vi "SMO.jsonRPC.Process.vi"(8 "error in (no error)":errorcluster, 11 "SMO.jsonRPC in":refnum<class "SMO.jsonRPC.lvclass">) -> (0 "error out":errorcluster)   [LabVIEW 2013, in "SMO.jsonRPC.lvclass"]
uses:
  SMO.jsonRPC.lvclass
  Typedefs/Request--Cluster.ctl
  <vilib>/JKI/JKI JSON RPC Specification/Request/Request.lvclass
  <vilib>/JKI/JKI JSON RPC Specification/Response/Response.lvclass
  <vilib>/JKI/JKI SMO/SMO/SMO.lvclass
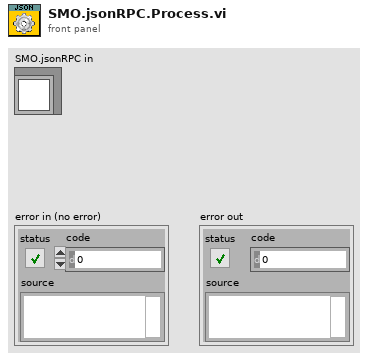
[diagram p1: front panel]
types:
  T1 = enum32{"invalid app kind", "Development System", "Run Time System", "Student Edition", "Embedded LabVIEW", "Evaluation", "Custom"}
  T2 = cluster{"Current VI Reference":refnum<vi>, "Close Panel on Exit?":bool, "error":errorcluster, "Standalone":bool}
  T3 = enum32{"Invalid", "Standard", "Closed", "Hidden", "Minimized", "Maximized"}
  T4 = typedef "SMO.jsonRPC.lvclass/Request--Cluster.ctl" = cluster{"Request":refnum<class "Request.lvclass">, "reply queue":refnum<queue>, "Async?":bool}
  T5 = cluster{"Core":cluster{"Current VI Reference":refnum<vi>, "Close Panel on Exit?":bool, "error":errorcluster, "Standalone":bool}, "Self Reference":refnum<class "SMO.jsonRPC.lvclass">, "Message Payload":T4}
  T6 = typedef "SMO.lvclass/SMOState --Enum.ctl" = enum16{"unknown", "Created", "Started", "Stopped"}
  T7 = typedef "SMO.lvclass/Protected Events.ctl" = cluster{"StopProcesses":refnum<user-event>, "AbortProcesses":refnum<user-event>, "Config Changed":refnum<user-event>}
  T8 = typedef "SMO.jsonRPC.lvclass/PrivateEvents--Cluster.ctl" = cluster{"Incoming Request":refnum<user-event>}
  T9 = typedef "SMO.jsonRPC.lvclass/PublicEvents--Cluster.ctl" = cluster{"Reply":refnum<user-event>}
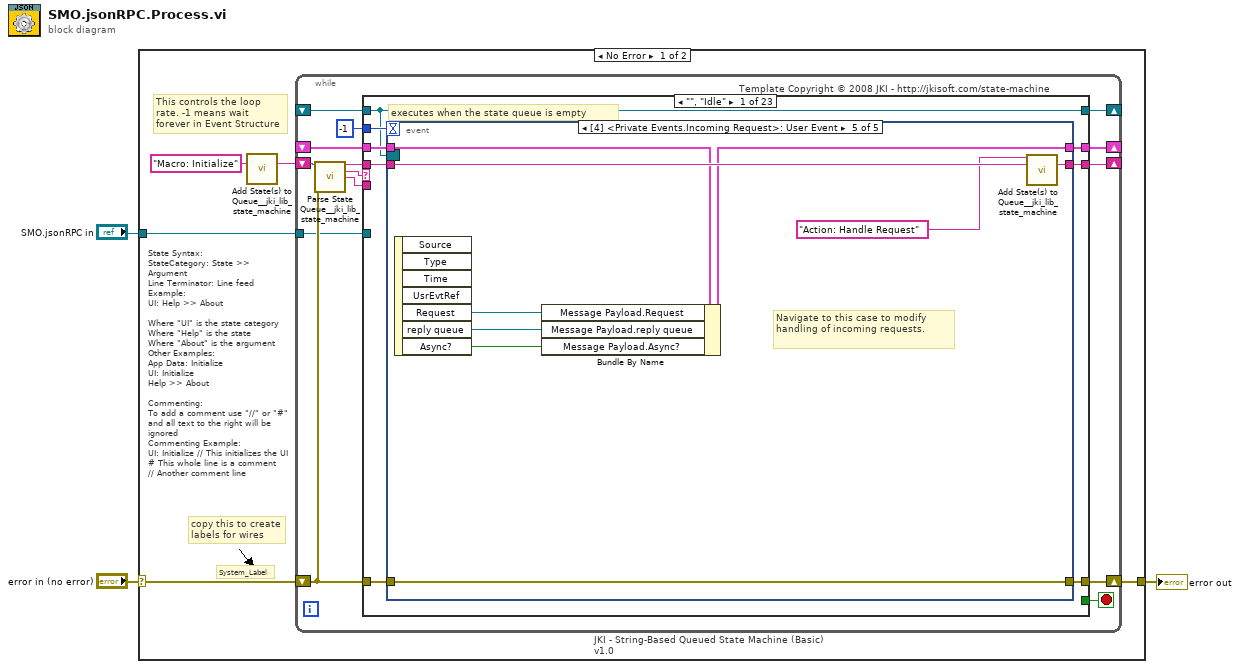
[diagram p0: block diagram]
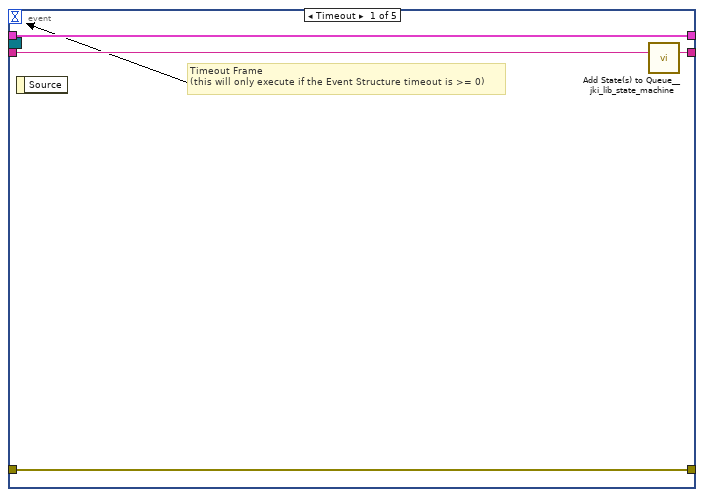
[diagram p2: hidden frame]
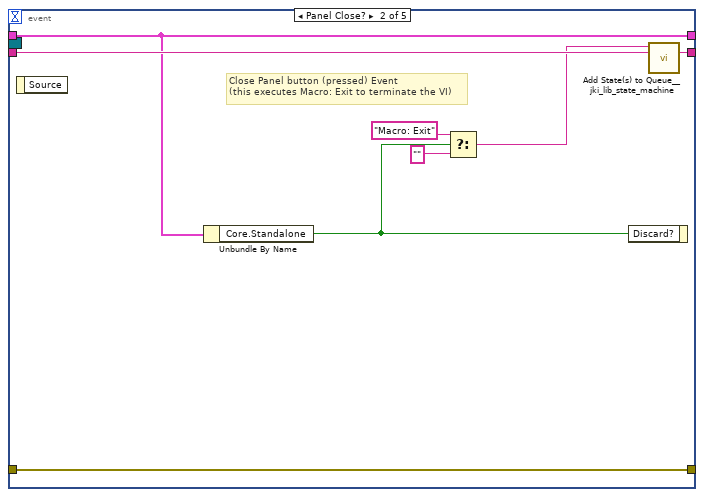
[diagram p3: hidden frame]
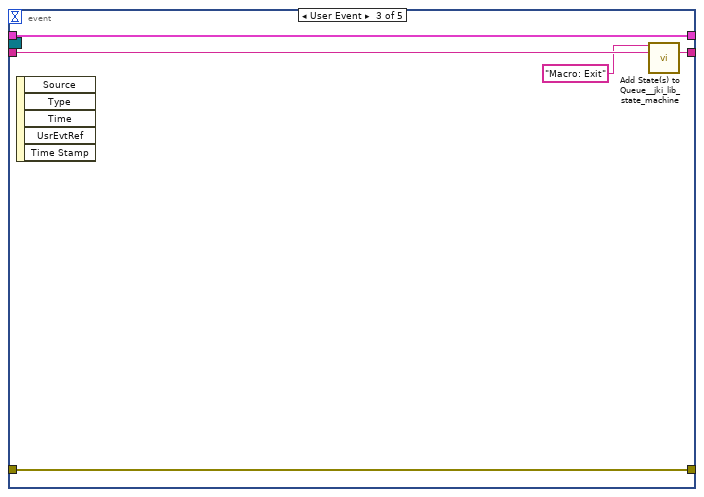
[diagram p4: hidden frame]
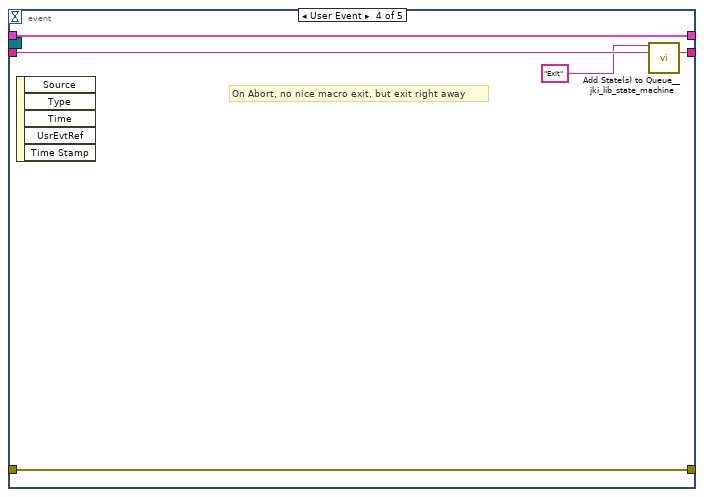
[diagram p5: hidden frame]
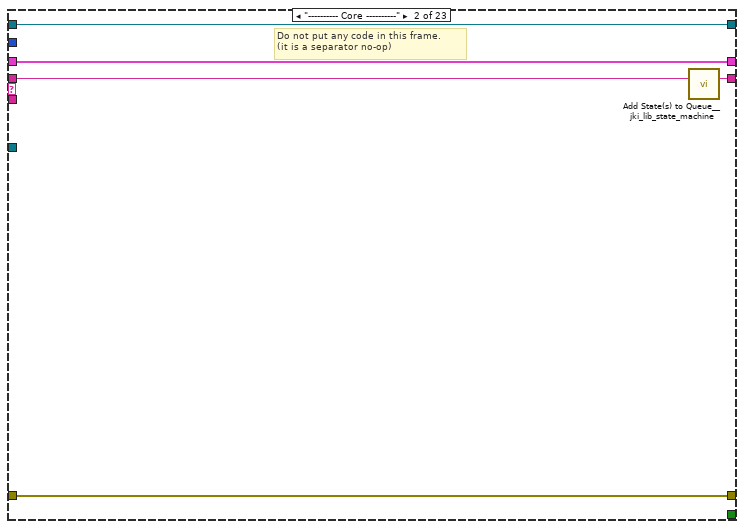
[diagram p6: hidden frame]
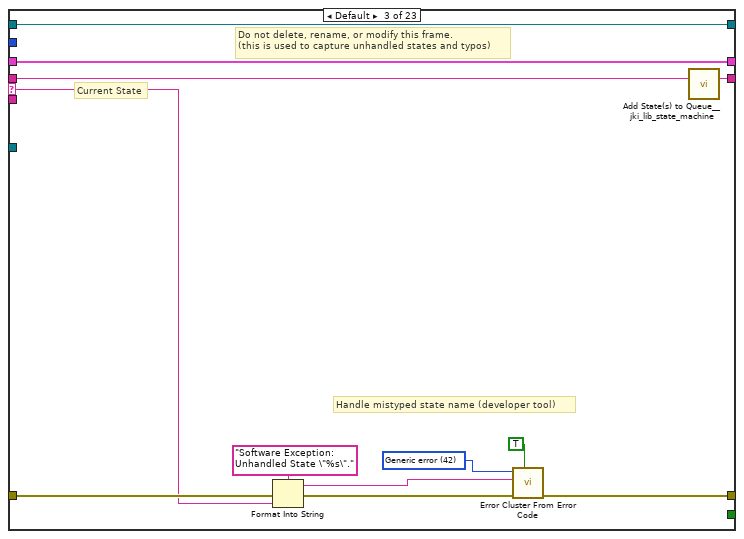
[diagram p7: hidden frame]
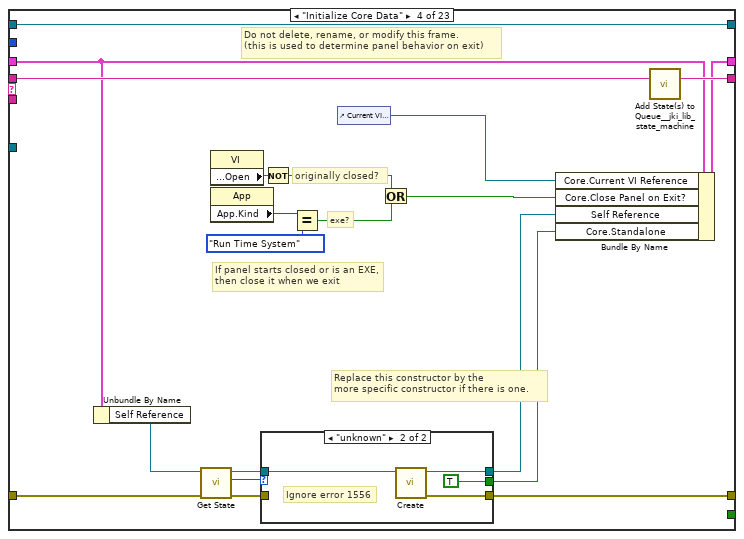
[diagram p8: hidden frame]
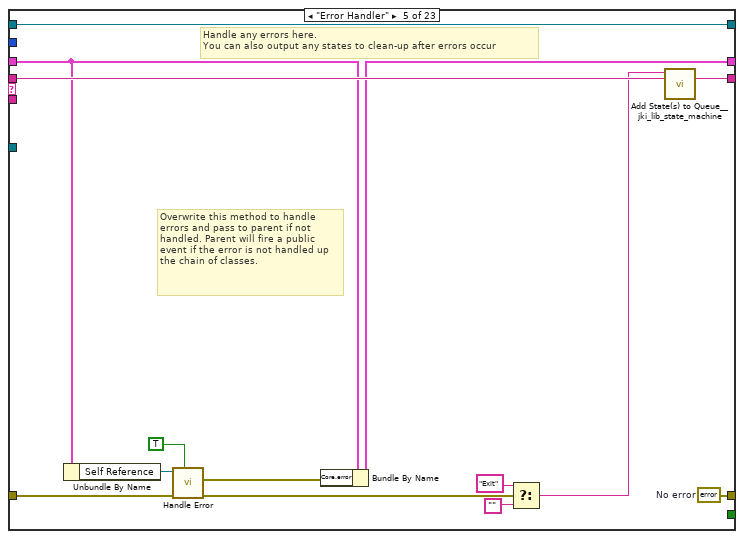
[diagram p10: hidden frame]
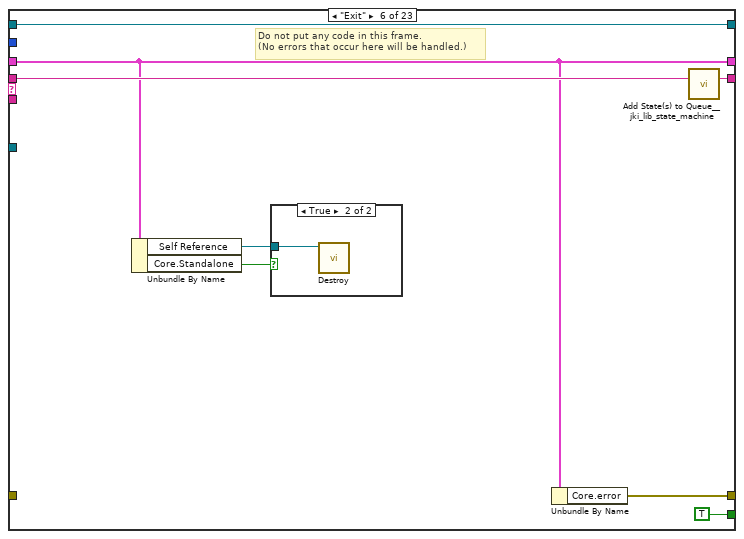
[diagram p11: hidden frame]
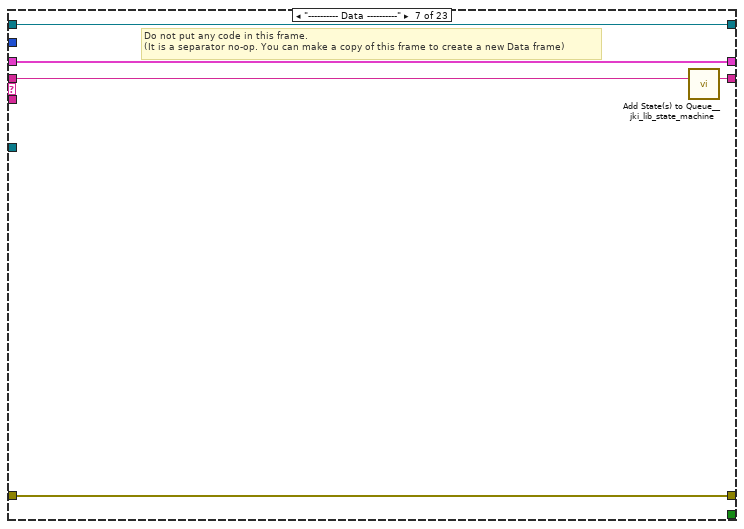
[diagram p13: hidden frame]
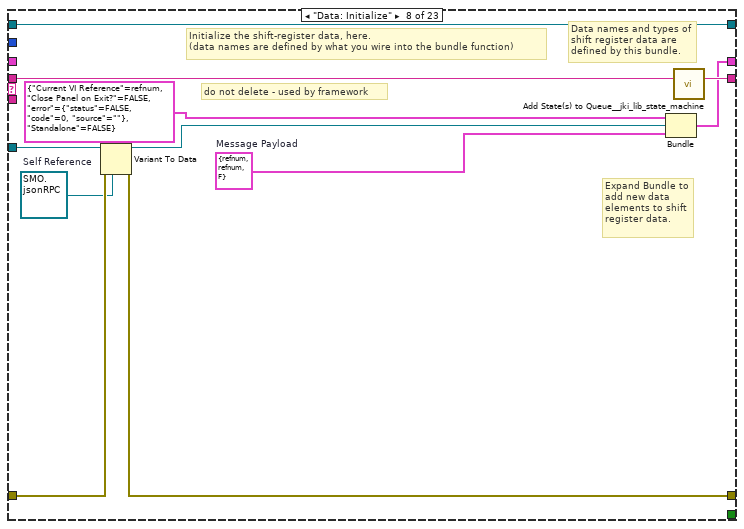
[diagram p14: hidden frame]
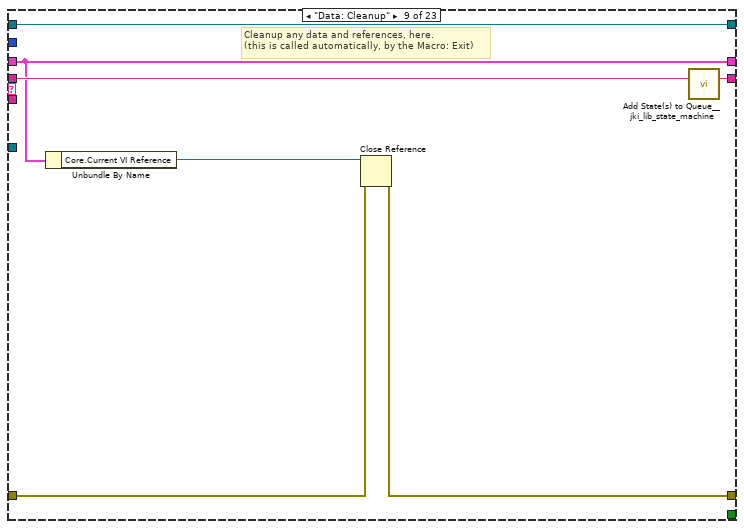
[diagram p15: hidden frame]
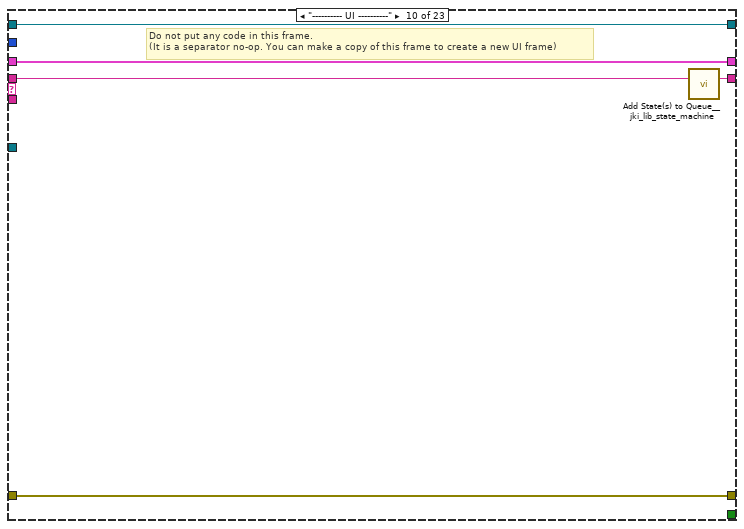
[diagram p16: hidden frame]
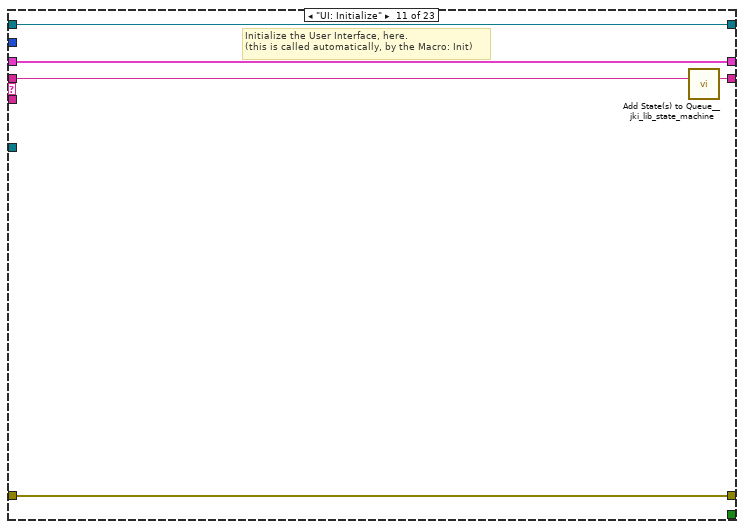
[diagram p17: hidden frame]
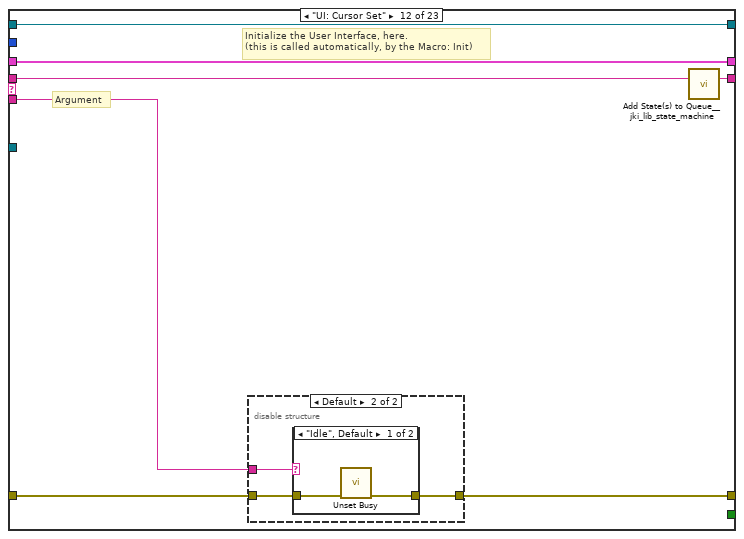
[diagram p18: hidden frame]
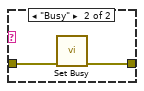
[diagram p20: hidden frame]
diagram:
  n1 = case shown="No Error" "error in (no error)" {
    selector: "error in (no error)" -> [w5 w304]
    tunnel: "SMO.jsonRPC in" -> [w6 _]
    tunnel: [w4 w304] -> w3
    frame No Error {
      # "State Syntax:\nStateCategory: State >> Argument\nLine Terminator: Line feed\nExample:\nUI: Help >> About\n\nWhere \"UI\" is the state category\nWhere \"Help\" is the state\nWhere \"About\" is the argument\nOther Examples:\nApp Data: Initialize\nUI: Initialize\nHelp >> About\n\nCommenting:\nTo add a comment use \"//\" or \"#\" and all text to the right will be ignored\nCommenting Example:\nUI: Initialize // This initializes the UI\n# This whole line is a comment\n// Another comment line"
      # "copy this to create labels for wires"
      # "This controls the loop rate. -1 means wait forever in Event Structure"
      # "System_Label"
      n2 = call <vilib>:"Add State(s) to Queue__jki_lib_state_machine.vi"("State(s) in (\"\")"="Macro: Initialize") -> ("States Out"=w8:string)  [unwired: 14 in]
      n3 = while "JKI - String-Based Queued State Machine (Basic) v1.0" {
        shift-right: [w15] -> _
        shift-left: _ -> [w14]
        shift-right: [w18] -> w4
        shift-left: w5 -> [w12]
        shift-right: [w17] -> _
        shift-left: w8 -> [w19]
        tunnel: w6 -> [w11]
        shift-right: [w10] -> _
        shift-left: _ -> [w9]
        stop <- w16 stop-if-true
        # "Template Copyright © 2008 JKI - http://jkisoft.com/state-machine"
        n4 = call <vilib>:"Parse State Queue__jki_lib_state_machine.vi"("State Queue"=w19, "Error In (no error)"=w12) -> ("Remaining States"=w21:string, "Current State"=w22:string, "Arguments"=w20:string)  [unwired: 11 in]
        n5 = case shown="\"\", \"Idle\"" w22 {
          selector: w22 -> [_ _ w68 _ _ _ _ _ _ _ _ _ _ _ _ _ _ _ _ _ _ _ _]
          tunnel: w21 -> [w30 w66 w72 w98 w118 w126 w132 w143 w150 w155 w160 w167 w183 w215 w221 w232 w237 w246 w259 w272 w278 w283 w299]
          tunnel: w20 -> [_ _ _ _ _ _ _ _ _ _ _ w161 w177 _ _ _ _ _ _ _ _ _ _]
          tunnel: w14 -> [w28 w63 w70 w82 w107 w119 w129 _ w145 w152 w158 w165 w179 w212 w217 w223 w234 w243 w256 w270 w276 w281 w296]
          tunnel: [w27 w64 w74 w81 w109 w122 w130 w139 w146 w153 w157 w162 w180 w213 w219 w230 w235 w240 w257 w260 w274 w279 w285] -> w18
          tunnel: w12 -> [w26 w64 w73 w83 w114 _ w130 w140 w147 w153 w157 w163 w181 w213 w219 w230 w235 w241 w257 w264 w274 w279 w294]
          tunnel: [w29 w65 w71 w97 w117 w125 w131 w142 w149 w154 w159 w166 w182 w214 w220 w231 w236 w245 w258 w271 w277 w282 w298] -> w17
          tunnel: [_ _ _ _ _ TRUE _ _ _ _ _ _ _ _ _ _ _ _ _ _ _ _ _] -> w16
          tunnel: [w25 w63 w70 w96 w106 w119 w129 w141 w145 w152 w158 w165 w179 w212 w217 w223 w234 w243 w256 w270 w276 w281 w296] -> w15
          tunnel: -1 ("Timeout") -> [w24 _ _ _ _ _ _ _ _ _ _ _ _ _ _ _ _ _ _ _ _ _ _]
          tunnel: w11 -> [_ _ _ _ _ _ _ w137 _ _ _ _ _ _ _ _ _ _ _ _ _ _ _]
          tunnel: [w23 w62 w67 w89 w116 w123 w128 w135 w144 w151 w156 w164 w176 w211 w218 w224 w233 w244 w255 w269 w275 w280 w297] -> w10
          tunnel: w9 -> [w23 w62 w67 w89 w116 w123 w128 w135 w144 w151 w156 w164 w176 w211 w218 w224 w233 w244 w255 _ w275 w280 w297]
          frame "", "Idle" {
            # "executes when the state queue is empty"
            n6 = event shown="[4] <Private Events.Incoming Request>: User Event" {
              selector: w23 -> [_ _ _ _ _]
              dyn-events: _ -> [_ _ _ _ _]
              timeout: w24 -> [_ _ _ _ _]
              tunnel: w30 -> [w34 w42 w47 w52 w61]
              tunnel: [w33 w41 w46 w51 w60] -> w29
              tunnel: w28 -> [w31 w37 w44 w49 w58]
              tunnel: [w32 w40 w45 w50 w59] -> w27
              tunnel: w26 -> [w32 w40 w45 w50 w59]
              tunnel: [w31 w37 w44 w49 w57] -> w25
              event Timeout {
                # "Timeout Frame\n(this will only execute if the Event Structure timeout is >= 0)"
                n7 = event-data() -> ()  [unwired: 1 in, 1 out]
                n8 = call <vilib>:"Add State(s) to Queue__jki_lib_state_machine.vi"("State(s) in (\"\")"=w34) -> ("States Out"=w33:string)  [unwired: 14 in]
              }
              event Panel Close? {
                # "Close Panel button (pressed) Event\n(this executes Macro: Exit to terminate the VI)"
                n9 = event-data() -> ()  [unwired: 1 in, 1 out]
                n10 = Unbundle By Name(w37) -> ("Core.Standalone"=w36:bool)
                n11 = Select(t="Macro: Exit", s=w36, f="") -> (s? t:f=w35:string)
                n12 = event-data("Discard?"=w36) -> ()  [unwired: 1 in, 1 out]
                n13 = call <vilib>:"Add State(s) to Queue__jki_lib_state_machine.vi"("State(s) in Front (\"\")"=w35, "State(s) in (\"\")"=w42) -> ("States Out"=w41:string)  [unwired: 13 in]
              }
              event User Event {
                n14 = event-data() -> ()  [unwired: 1 in, 5 out]
                n15 = call <vilib>:"Add State(s) to Queue__jki_lib_state_machine.vi"("State(s) in Front (\"\")"="Macro: Exit", "State(s) in (\"\")"=w47) -> ("States Out"=w46:string)  [unwired: 13 in]
              }
              event User Event {
                # "On Abort, no nice macro exit, but exit right away"
                n16 = event-data() -> ()  [unwired: 1 in, 5 out]
                n17 = call <vilib>:"Add State(s) to Queue__jki_lib_state_machine.vi"("State(s) in Front (\"\")"="Exit", "State(s) in (\"\")"=w52) -> ("States Out"=w51:string)  [unwired: 13 in]
              }
              event User Event {
                # "Navigate to this case to modify handling of incoming requests."
                n18 = event-data() -> ("Request"=w55:refnum<class "Request.lvclass">, "reply queue"=w54:refnum<queue>, "Async?"=w53:bool)  [unwired: 1 in, 4 out]
                n19 = Bundle By Name(cluster=w58, "Message Payload.Request"=w55, "Message Payload.reply queue"=w54, "Message Payload.Async?"=w53) -> (w57:T5)
                n20 = call <vilib>:"Add State(s) to Queue__jki_lib_state_machine.vi"("State(s) in Front (\"\")"="Action: Handle Request", "State(s) in (\"\")"=w61) -> ("States Out"=w60:string)  [unwired: 13 in]
              }
            }
          }
          frame "---------- Core ----------" {
            # "Do not put any code in this frame.\n(it is a separator no-op)"
            n21 = call <vilib>:"Add State(s) to Queue__jki_lib_state_machine.vi"("State(s) in (\"\")"=w66) -> ("States Out"=w65:string)  [unwired: 14 in]
          }
          frame Default {
            w77 = 42 items=["No error", "Argument error", "Memory is full", "Out of zone", "End of file", "File already open", "Generic file I/O error", "File not found", "File permission error", "Disk is full", "Duplicate path", "Too many files open", "System feature not enabled", "Resource file not found", "Cannot add resource", "Resource not found", "Image not found", "Image memory error", "Pen does not exist", "Config type invalid", "Config token not found", "Config parse error", "Config memory error", "Bad external code format", "Bad external code offset", "External code not present", "Null window", "Destroy window error", "Null menu", "Print aborted", "Bad print record", "Print driver error", "Windows error during printing", "Memory error during printing", "Print dialog error", "Generic print error", "Invalid device refnum", "Device not found", "Device parameter error", "Device unit error", "Cannot open device", "Device call aborted", "Generic error", "Cancelled by user", "Object ID too low", "Object ID too high", "Object not in heap", "Unknown heap", "Unknown object (invalid DefProc)", "Unknown object (DefProc not in table)", "Message out of range", "Invalid (null) method", "Unknown message", "Manager call not supported", "Bad address", "Network operation in progress", "Network operation timed out", "Connection is busy", "Network attribute not supported", "Network error", "Address in use", "System out of memory", "Connection aborted", "Connection refused", "Not connected", "Already connected", "Connection closed", "Initialization error (interapplication manager)", "Bad occurrence", "Wait on unbound occurrence handler", "Occurrence queue overflow", "Datalog type conflict", "Unused", "Unrecognized type (interapplication manager)", "Memory corrupt", "Failed to make temporary DLL", "Old CIN version", "Drag socket not found", "Failed to load drop-object", "Failed to register OLE object", "Failed to release OLE object", "Format specifier type mismatch", "Unknown format specifier", "Too few format specifiers", "Too many format specifiers", "Scan failed", "Newer CIN version", "Error converting to variant", "Runtime menu error", "Password tampered", "Variant attribute not found", "Incompatible variant data type", "Event data is not available", "Event Store is not present", "Occurrence is not found", "Event Queue is not created", "Event info is not available", "Refnum passed is NULL", "Error retrieving Class GUID", "Error retrieving CoClass GUID", "Error retrieving TypeLib GUID.", "Bad built application magic bytes.", "Specific driver is different from the specific driver associated with the Logical Name.", "There is no session opened to the class driver.", "Max Error", "MAX - Error with config objects", "MAX - Error loading configuration", "MAX - Group not supported"]
            # "Current State"
            # "Do not delete, rename, or modify this frame.\n(this is used to capture unhandled states and typos)"
            # "Handle mistyped state name (developer tool)"
            n22 = Format Into String(format string="Software Exception: Unhandled State \"%s\"." ("message"), error in=w73, w68) -> (resulting string=w76:string, error out=w75:errorcluster)  [unwired: 1 in]
            n23 = call <vilib>:"Error Cluster From Error Code.vi"("show call chain? (False)"=TRUE, "error in (no error)"=w75, "error message (\"\")"=w76, "error code (0)"=w77) -> ("error out"=w74:errorcluster)  [unwired: 5 in]
            n24 = call <vilib>:"Add State(s) to Queue__jki_lib_state_machine.vi"("State(s) in (\"\")"=w72) -> ("States Out"=w71:string)  [unwired: 14 in]
          }
          frame "Initialize Core Data" {
            # "Replace this constructor by the\nmore specific constructor if there is one."
            # "Do not delete, rename, or modify this frame.\n(this is used to determine panel behavior on exit)"
            # "originally closed?"
            # "exe?"
            # "If panel starts closed or is an EXE, then close it when we exit"
            n25 = Unbundle By Name(w82) -> ("Self Reference"=w87:refnum<class "SMO.jsonRPC.lvclass">)
            n26 = call <vilib>:"Get State.vi"("error in (no error)"=w83, "SMO"=w87) -> ("error out"=w85:errorcluster, "SMO State"=w84:T6, "SMO out"=w86:refnum<class "SMO.jsonRPC.lvclass">)  [unwired: 7 in]
            n27 = property class="VI"() -> ("Front Panel.Open"=w95:bool)  [unwired: 2 in, 2 out]
            n28 = property class="App"() -> ("App.Kind"=w94:T1)  [unwired: 2 in, 2 out]
            n29 = case shown="\"unknown\"" w84 {
              tunnel: w86 -> [w100 w104]
              tunnel: w85 -> [w99 _]
              tunnel: [w99 w103] -> w81
              tunnel: [w100 w102] -> w80
              tunnel: [_ TRUE] -> w79
              frame Default {
              }
              frame "unknown" {
                # "Ignore error 1556"
                n30 = call <vilib>:"Create.vi"("SMO"=w104) -> ("error out"=w103:errorcluster, "SMO out"=w102:refnum<class "SMO.jsonRPC.lvclass">)  [unwired: 8 in, 1 out]
              }
            }
            n31 = Not(x=w95) -> (.not. x?=w92:bool)
            n32 = Equal?(x=w94, y=T1."Run Time System" ("Application:Kind")) -> (x = y?=w91:bool)
            n33 = control-ref of="Current VI Reference"() -> (w88:refnum<vi>)
            n34 = Or(x=w92, y=w91) -> (x .or. y?=w90:bool)
            n35 = Bundle By Name(cluster=w82, "Core.Current VI Reference"=w88, "Core.Close Panel on Exit?"=w90, "Self Reference"=w80, "Core.Standalone"=w79) -> (w96:T5)
            n36 = call <vilib>:"Add State(s) to Queue__jki_lib_state_machine.vi"("State(s) in (\"\")"=w98) -> ("States Out"=w97:string)  [unwired: 14 in]
          }
          frame "Error Handler" {
            w109 = errorcluster {"status"=FALSE, "code"=0, "source"=""}  # No error
            # "Overwrite this method to handle errors and pass to parent if not handled. Parent will fire a public event if the error is not handled up the chain of classes."
            # "Handle any errors here.\nYou can also output any states to clean-up after errors occur"
            n37 = Unbundle By Name(w107) -> ("Self Reference"=w115:refnum<class "SMO.jsonRPC.lvclass">)
            n38 = call-dynamic "Handle Error.vi"("Stop on Unhandled Error (T)"=TRUE, "error in"=w114, "SMO"=w115) -> ("handling error"=w110:errorcluster, "Unhandled error"=w108:errorcluster)  [unwired: 6 in, 1 out]
            n39 = Bundle By Name(cluster=w107, "Core.error"=w108) -> (w106:T5)
            n40 = Select(t="Exit", s=w110, f="") -> (s? t:f=w111:string)
            n41 = call <vilib>:"Add State(s) to Queue__jki_lib_state_machine.vi"("State(s) in Front (\"\")"=w111, "State(s) in (\"\")"=w118) -> ("States Out"=w117:string)  [unwired: 13 in]
          }
          frame "Exit" {
            # "Do not put any code in this frame.\n(No errors that occur here will be handled.)"
            n42 = Unbundle By Name(w119) -> ("Self Reference"=w121:refnum<class "SMO.jsonRPC.lvclass">, "Core.Standalone"=w120:bool)
            n43 = case shown="True" w120 {
              tunnel: w121 -> [_ w127]
              frame False {
              }
              frame True {
                n44 = call <vilib>:"Destroy.vi"("SMO"=w127) -> ()  [unwired: 10 in, 1 out]
              }
            }
            n45 = Unbundle By Name(w119) -> ("Core.error"=w122:errorcluster)
            n46 = call <vilib>:"Add State(s) to Queue__jki_lib_state_machine.vi"("State(s) in (\"\")"=w126) -> ("States Out"=w125:string)  [unwired: 14 in]
          }
          frame "---------- Data ----------" {
            # "Do not put any code in this frame.\n(It is a separator no-op. You can make a copy of this frame to create a new Data frame)"
            n47 = call <vilib>:"Add State(s) to Queue__jki_lib_state_machine.vi"("State(s) in (\"\")"=w132) -> ("States Out"=w131:string)  [unwired: 14 in]
          }
          frame "Data: Initialize" {
            w133 = T4 {"Request"=refnum, "reply queue"=refnum, "Async?"=FALSE}  # Message Payload
            w138 = refnum<class "SMO.jsonRPC.lvclass"> refnum  # Self Reference
            # "do not delete - used by framework"
            # "Expand Bundle to add new data elements to shift register data."
            # "Data names and types of shift register data are defined by this bundle."
            # "Initialize the shift-register data, here.\n(data names are defined by what you wire into the bundle function)"
            n48 = Variant To Data(error in=w140, type=w138, Variant=w137) -> (data=w136:refnum<class "SMO.jsonRPC.lvclass">, error out=w139:errorcluster)
            n49 = Bundle("Core"=T2 {"Current VI Reference"=refnum, "Close Panel on Exit?"=FALSE, "error"={"status"=FALSE, "code"=0, "source"=""}, "Standalone"=FALSE}, "Self Reference"=w136, "Message Payload"=w133) -> (w141:T5)  [unwired: 1 in]
            n50 = call <vilib>:"Add State(s) to Queue__jki_lib_state_machine.vi"("State(s) in (\"\")"=w143) -> ("States Out"=w142:string)  [unwired: 14 in]
          }
          frame "Data: Cleanup" {
            # "Cleanup any data and references, here.\n(this is called automatically, by the Macro: Exit)"
            n51 = Unbundle By Name(w145) -> ("Core.Current VI Reference"=w148:refnum<vi>)
            n52 = Close Reference(reference=w148, error in (no error)=w147) -> (error out=w146:errorcluster)
            n53 = call <vilib>:"Add State(s) to Queue__jki_lib_state_machine.vi"("State(s) in (\"\")"=w150) -> ("States Out"=w149:string)  [unwired: 14 in]
          }
          frame "---------- UI ----------" {
            # "Do not put any code in this frame.\n(It is a separator no-op. You can make a copy of this frame to create a new UI frame)"
            n54 = call <vilib>:"Add State(s) to Queue__jki_lib_state_machine.vi"("State(s) in (\"\")"=w155) -> ("States Out"=w154:string)  [unwired: 14 in]
          }
          frame "UI: Initialize" {
            # "Initialize the User Interface, here.\n(this is called automatically, by the Macro: Init)"
            n55 = call <vilib>:"Add State(s) to Queue__jki_lib_state_machine.vi"("State(s) in (\"\")"=w160) -> ("States Out"=w159:string)  [unwired: 14 in]
          }
          frame "UI: Cursor Set" {
            # "Argument"
            # "Initialize the User Interface, here.\n(this is called automatically, by the Macro: Init)"
            n56 = disable-structure shown="Default" {
              disable-tunnel: w163 -> [w168 w171]
              disable-tunnel: [w168 w170] -> w162
              disable-tunnel: w161 -> [_ w169]
              frame condition #0 {
              }
              frame condition #1 (active) {
                n57 = case shown="\"Idle\", Default" w169 {
                  tunnel: w171 -> [w173 w175]
                  tunnel: [w172 w174] -> w170
                  frame "Idle", Default {
                    n58 = call <vilib>:"Unset Busy.vi"("error in (no error)"=w173) -> ("error out"=w172:errorcluster)  [unwired: 10 in]
                  }
                  frame "Busy" {
                    n59 = call <vilib>:"Set Busy.vi"("error in (no error)"=w175) -> ("error out"=w174:errorcluster)  [unwired: 9 in, 1 out]
                  }
                }
              }
            }
            n60 = call <vilib>:"Add State(s) to Queue__jki_lib_state_machine.vi"("State(s) in (\"\")"=w167) -> ("States Out"=w166:string)  [unwired: 14 in]
          }
          frame "UI: Front Panel State" {
            # "Argument"
            # "Set Front Panel Open or Closed\n(Usage: \"UI: Front Panel State >> Open|Close\")"
            n61 = Unbundle By Name(w179) -> ("Core.Current VI Reference"=w178:refnum<vi>)
            n62 = disable-structure shown="Default" {
              disable-tunnel: w181 -> [w187 w210]
              disable-tunnel: [w186 w210] -> w180
              disable-tunnel: w178 -> [w185 _]
              disable-tunnel: w177 -> [w184 _]
              frame condition #0 (active) {
                n63 = case shown="\"Close\"" w184 {
                  tunnel: w187 -> [w191 w204]
                  tunnel: [w193 w205] -> w186
                  tunnel: w185 -> [w192 w202]
                  frame "Open", Default {
                    n64 = property class="VI"(reference=w192, error in=w191) -> (reference out=w189:refnum<vi>, error out=w190:errorcluster, "FP.State"=w188:T3)
                    n65 = case shown="\"Closed\"" w188 {
                      tunnel: [w196 w199] -> w193
                      tunnel: w190 -> [w195 w199]
                      tunnel: w189 -> [w194 _]
                      frame "Closed" {
                        n66 = invoke class="VI" method="FP.Open"(reference=w194, error in=w195, "Activate"=TRUE, "State"=T3."Standard") -> (error out=w196:errorcluster)  [unwired: 1 in, 4 out]
                      }
                      frame Default {
                      }
                    }
                  }
                  frame "Close" {
                    n67 = property class="VI"(reference=w202, error in=w204) -> (reference out=w201:refnum<vi>, error out=w203:errorcluster, "FP.State"=w200:T3)
                    n68 = case shown="Default" w200 {
                      tunnel: [w206 w209] -> w205
                      tunnel: w203 -> [w206 w208]
                      tunnel: w201 -> [_ w207]
                      frame "Invalid", "Closed" {
                      }
                      frame Default {
                        n69 = invoke class="VI" method="FP.Close"(reference=w207, error in=w208) -> (error out=w209:errorcluster)  [unwired: 1 in, 2 out]
                      }
                    }
                  }
                }
              }
              frame condition #1 {
              }
            }
            n70 = call <vilib>:"Add State(s) to Queue__jki_lib_state_machine.vi"("State(s) in (\"\")"=w183) -> ("States Out"=w182:string)  [unwired: 14 in]
          }
          frame "---------- Macro ----------" {
            # "Do not put any code in this frame.\n(It is a separator no-op. You can make a copy of this frame to create a new Macro frame)"
            n71 = call <vilib>:"Add State(s) to Queue__jki_lib_state_machine.vi"("State(s) in (\"\")"=w215) -> ("States Out"=w214:string)  [unwired: 14 in]
          }
          frame "Macro: Initialize" {
            # "Initialization Macro\n(This is called once, when the VI starts)"
            n72 = call <vilib>:"Add State(s) to Queue__jki_lib_state_machine.vi"("State(s) in Front (\"\")"="Data: Initialize\nInitialize Core Data\nEvents: Register\nProcess: Sync", "State(s) in (\"\")"=w221) -> ("States Out"=w220:string)  [unwired: 13 in]
          }
          frame "Macro: Exit" {
            # "Exit Macro\n(This is called once, when the VI exits)"
            n73 = Unbundle By Name(w223) -> ("Core.Close Panel on Exit?"=w229:bool)
            n74 = Select(t="UI: Front Panel State >> Close", s=w229, f="") -> (s? t:f=w226:string)
            n75 = call <vilib>:"Add State(s) to Queue__jki_lib_state_machine.vi"("State(s) in (\"\")"=w226, "State(s) at Back (\"\")"="Data: Cleanup\nEvents: Unregister\nProcess: Sync\nExit") -> ("States Out"=w225:string)  [unwired: 13 in]
            n76 = call <vilib>:"Add State(s) to Queue__jki_lib_state_machine.vi"("State(s) in Front (\"\")"=w225, "State(s) in (\"\")"=w232) -> ("States Out"=w231:string)  [unwired: 13 in]
          }
          frame "---------- Process ----------" {
            # "Template Separator\n(You can make a copy of, or modify, this frame)"
            n77 = call <vilib>:"Add State(s) to Queue__jki_lib_state_machine.vi"("State(s) in (\"\")"=w237) -> ("States Out"=w236:string)  [unwired: 14 in]
          }
          frame "Process: Sync" {
            n78 = Unbundle By Name(w243) -> ("Self Reference"=w242:refnum<class "SMO.jsonRPC.lvclass">, "Core.Standalone"=w238:bool)
            n79 = case shown="False" w238 {
              tunnel: w242 -> [w250 _]
              tunnel: w241 -> [w249 w254]
              tunnel: [w248 w254] -> w240
              tunnel: [w247 _] -> w239
              frame False {
                n80 = call <vilib>:"WaitOnProcessSync.vi"("error in (no error)"=w249, "SMO"=w250) -> ("error out"=w248:errorcluster, "Don't run?"=w253:bool)  [unwired: 7 in, 1 out]
                n81 = Select(t="Data: Cleanup\nEvents: Unregister\nExit", s=w253, f="") -> (s? t:f=w247:string)
              }
              frame True {
              }
            }
            n82 = call <vilib>:"Add State(s) to Queue__jki_lib_state_machine.vi"("State(s) in Front (\"\")"=w239, "State(s) in (\"\")"=w246) -> ("States Out"=w245:string)  [unwired: 13 in]
          }
          frame "---------- Events ----------" {
            # "Template Separator\n(You can make a copy of, or modify, this frame)"
            n83 = call <vilib>:"Add State(s) to Queue__jki_lib_state_machine.vi"("State(s) in (\"\")"=w259) -> ("States Out"=w258:string)  [unwired: 14 in]
          }
          frame "Events: Register" {
            # "Expand to add\nmore events"
            # "Self Events (API Calls)"
            # "Base Class Protected Events"
            n84 = Unbundle By Name(w270) -> ("Self Reference"=w265:refnum<class "SMO.jsonRPC.lvclass">)
            n85 = call <vilib>:"GetProtectedEvents.vi"("SMO"=w265) -> ("error out"=w261:errorcluster, "SMO Protected Events"=w268:T7, "SMO out"=w267:refnum<class "SMO.jsonRPC.lvclass">)  [unwired: 8 in]
            n86 = call "SMO.jsonRPC.GetPrivateEvents.vi"("SMO.jsonRPC"=w267) -> ("error out"=w262:errorcluster, "Private Events"=w266:T8)  [unwired: 8 in, 1 out]
            n87 = register-events(w268, w266) -> (reference out=w269:refnum<event-registration>, error out=w263:errorcluster)  [unwired: 2 in]
            n88 = Merge Errors(w264, w263, w262, w261) -> (w260:errorcluster)
            n89 = call <vilib>:"Add State(s) to Queue__jki_lib_state_machine.vi"("State(s) in (\"\")"=w272) -> ("States Out"=w271:string)  [unwired: 14 in]
          }
          frame "Events: Unregister" {
            n90 = Unregister For Events(event registration refnum=w275, error in=w274) -> (error out=w273:errorcluster)
            n91 = call <vilib>:"Clear Errors.vi"("error in (no error)"=w273) -> ()  [unwired: 6 in, 1 out]
            n92 = call <vilib>:"Add State(s) to Queue__jki_lib_state_machine.vi"("State(s) in (\"\")"=w278) -> ("States Out"=w277:string)  [unwired: 14 in]
          }
          frame "---------- Action ----------" {
            n93 = call <vilib>:"Add State(s) to Queue__jki_lib_state_machine.vi"("State(s) in (\"\")"=w283) -> ("States Out"=w282:string)  [unwired: 14 in]
          }
          frame "Action: Handle Request" {
            # "Edit this method to handle all the\ndifferent messages."
            n94 = Unbundle By Name(w296) -> ("Message Payload.reply queue"=w293:refnum<queue>, "Message Payload.Async?"=w292:bool, "Self Reference"=w288:refnum<class "SMO.jsonRPC.lvclass">, "Message Payload.Request"=w295:refnum<class "Request.lvclass">)
            n95 = call "HandleJsonRpcRequest.vi"("error in (no error)"=w294, "Request"=w295, "SMO.jsonRPC"=w288) -> ("error out"=w286:errorcluster, "Response"=w284:refnum<class "Response.lvclass">, "SMO.jsonRPC out"=w287:refnum<class "SMO.jsonRPC.lvclass">)  [unwired: 6 in]
            n96 = call "SMO.jsonRPC.GetPublicEvents.vi"("error in (no error)"=w286, "SMO.ByRefWithEvents"=w287) -> ("error out"=w291:errorcluster, "SMO.ByRefWithEvents Public Events"=w289:T9)  [unwired: 7 in, 1 out]
            n97 = Unbundle By Name(w289) -> ("Reply"=w290:refnum<user-event>)
            n98 = Generate User Event(user event=w290, event data cluster=w284, error in=w291) -> (error out=w285:errorcluster)  [unwired: 1 in, 1 out]
            n99 = case shown="False" w292 {
              tunnel: w293 -> [w303 _]
              tunnel: w284 -> [w302 _]
              frame False {
                n100 = Enqueue Element(queue=w303, element=w302, timeout in ms (-1)=0) -> (error out=w300:errorcluster)  [unwired: 1 in, 2 out]
                n101 = call <vilib>:"Clear Errors.vi"("error in (no error)"=w300) -> ()  [unwired: 6 in, 1 out]
              }
              frame True {
              }
            }
            n102 = call <vilib>:"Add State(s) to Queue__jki_lib_state_machine.vi"("State(s) in (\"\")"=w299) -> ("States Out"=w298:string)  [unwired: 14 in]
          }
        }
      }
    }
    frame Error {
    }
  }
  "error out" <- w3
